vi "Incrementer.vi"(1 "N":i32, 7 "reset":bool) -> (8 "Count":i32)   [LabVIEW 2016]
panel:
  out "x-y*floor(x/y)":i32
  out "x*y":i32
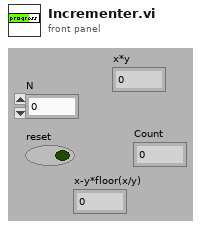
[diagram p1: front panel]
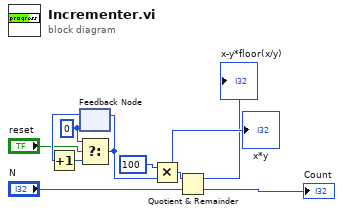
[diagram p0: block diagram]
diagram:
  w8 = 0
  n1 = feedback #1(w8) -> (w10:i32)
  n2 = Increment(x=w10) -> (x+1=w7:i32)
  n3 = Select(t=w8, s="reset", f=w7) -> (s? t:f=w3:i32)
  n4 = feedback-in #1(w3) -> ()
  n5 = Multiply(x=100, y=w3) -> (x*y=w6:i32)
  "x*y" <- w6
  n6 = Quotient & Remainder(x=w6, y="N") -> (x-y*floor(x/y)=→"x-y*floor(x/y)":i32, floor(x/y)=→"Count":i32)
